vi "RDS Serial Handler Read.vi"(8 "error in (no error)":errorcluster, 11 "RDS Serial Instrument in":refnum<class "RDS Serial Instrument.lvclass">) -> (0 "error out":errorcluster, 1 "Data Valid?":bool, 2 "RDS Serial Frame out":refnum<class "RDS Serial Frame.lvclass">, 3 "RDS Serial Instrument out":refnum<class "RDS Serial Instrument.lvclass">)   [LabVIEW 2015, in "RDS Serial Handler.lvlib" / "RDS Serial Instrument.lvclass"]
doc: "Neat little program that reads the serial port and looks for a set of termination characters. The reason for this is that labview's serial functions only accept ONE termination character, meaning that I'll have to do lots of work arounds to use it, so might as well make my own clean implementation. \n\nThis VI reads data from a serial port untill it times out or it finds the termination character."
uses:
  RDS Serial Instrument.lvclass
  RDS Serial Frame.lvclass
  RDS Serial Instrument.lvclass/RDS Serial Instrument.ctl
  RDS Serial Frame.lvclass/RDS Serial Frame.ctl
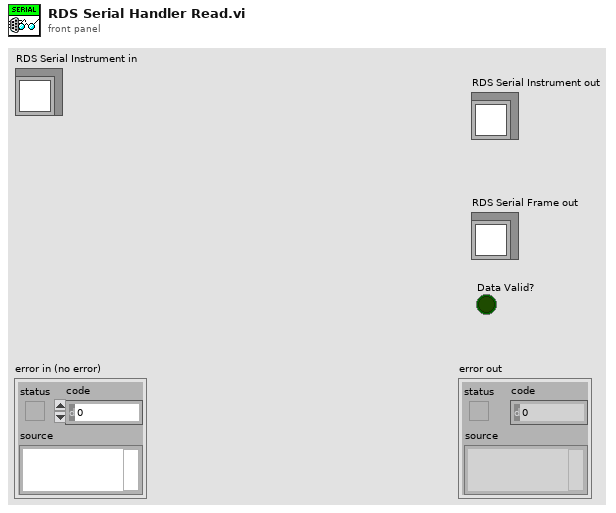
[diagram p1: front panel]
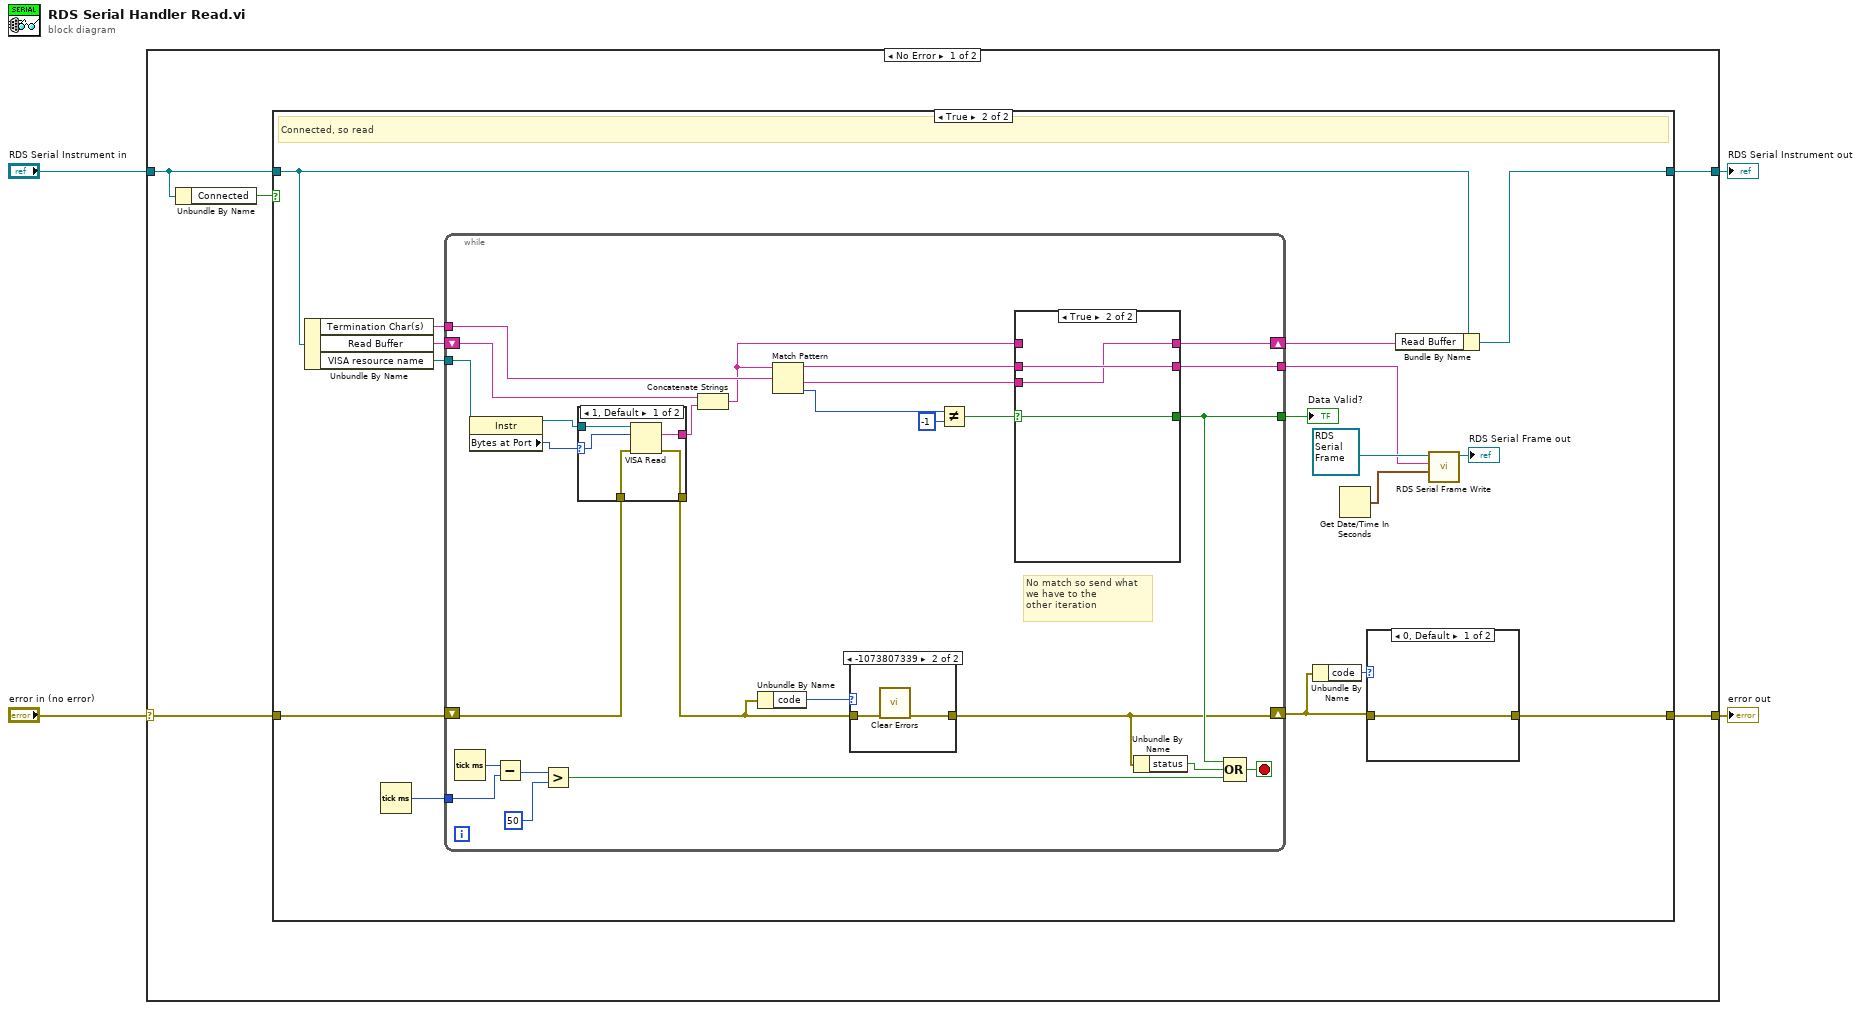
[diagram p0: block diagram]
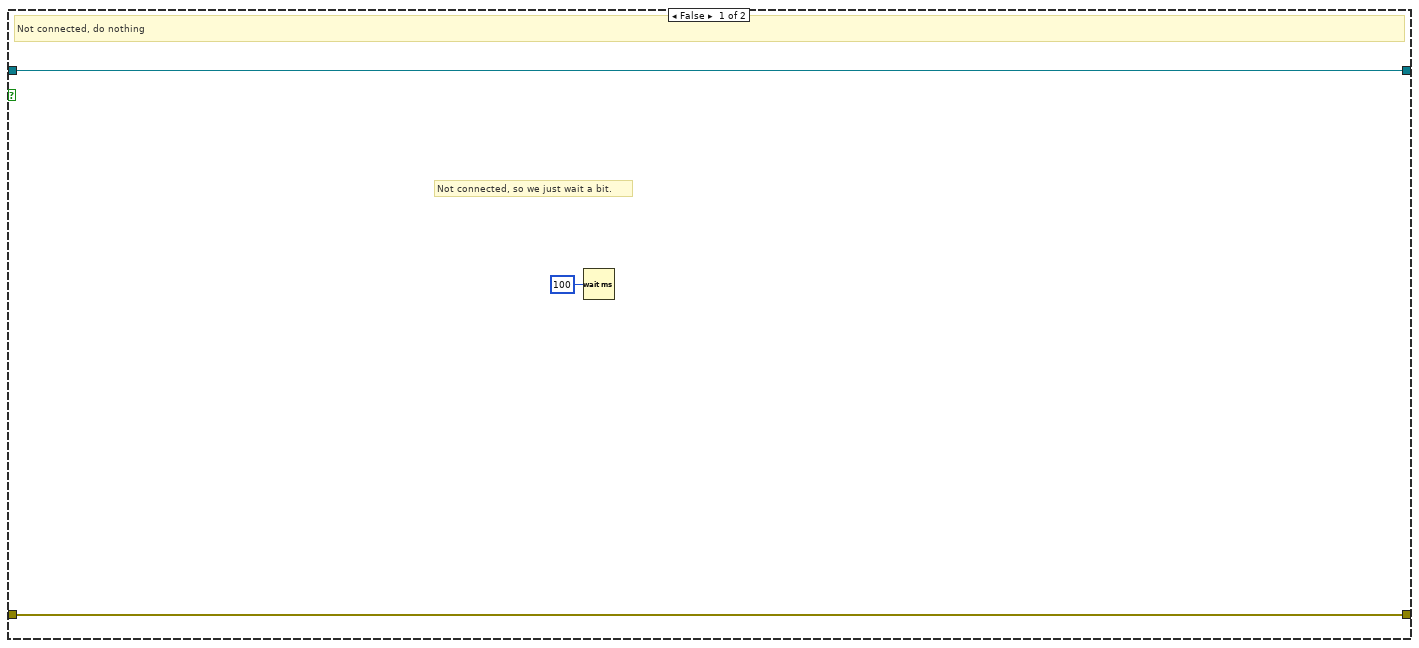
[diagram p2: hidden frame]
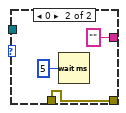
[diagram p3: hidden frame]
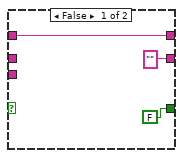
[diagram p4: hidden frame]
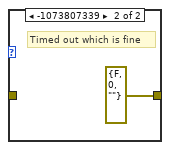
[diagram p6: hidden frame]
diagram:
  n1 = case shown="No Error" "error in (no error)" {
    selector: "error in (no error)" -> [w9 w75]
    tunnel: [w8 w75] -> w3
    tunnel: [w7 w74] -> w1
    tunnel: "RDS Serial Instrument in" -> [w6 w74]
    frame No Error {
      n2 = Unbundle By Name(w6) -> ("Connected"=w5:bool)
      n3 = case shown="True" w5 {
        tunnel: w9 -> [w11 w28]
        tunnel: [w11 w21] -> w8
        tunnel: w6 -> [w12 w20]
        tunnel: [w12 w19] -> w7
        frame False {
          # "Not connected, so we just wait a bit."
          # "Not connected, do nothing"
          n4 = Wait (ms)(milliseconds to wait=u32 100) -> ()  [unwired: 1 out]
        }
        frame True {
          # "Connected, so read"
          n5 = Unbundle By Name(w20) -> ("Termination Char(s)"=w25:string, "Read Buffer"=w27:string, "VISA resource name"=w26:refnum<visa-resource-name>)
          n6 = Tick Count (ms)() -> (millisecond timer value=w18:u32)
          n7 = while {
            tunnel: w26 -> [w38]
            tunnel: w25 -> [w51]
            tunnel: [w45] -> w24
            shift-right: [w39] -> w22
            shift-left: w28 -> [w54]
            shift-right: [w53] -> w16
            shift-left: w27 -> [w52]
            tunnel: [w50] -> w13
            tunnel: w18 -> [w48]
            stop <- w42 stop-if-true
            # "No match so send what\nwe have to the \nother iteration"
            n8 = Tick Count (ms)() -> (millisecond timer value=w49:u32)
            n9 = property class="Instr"(reference=w38) -> (reference out=w37:refnum<visa-resource-name>, "Bytes at Port"=w29:u32)  [unwired: 1 in, 1 out]
            n10 = Subtract(x=w49, y=w48) -> (x-y=w47:u32)
            n11 = Greater?(x=w47, y=u32 50) -> (0:w44:bool)
            n12 = case shown="1, Default" w29 {
              selector: w29 -> [w55 _]
              tunnel: w54 -> [w59 w60]
              tunnel: [w58 w60] -> w41
              tunnel: w37 -> [w57 _]
              tunnel: [w56 "" ("read buffer")] -> w30
              frame 1, Default {
                n13 = VISA Read(VISA resource name=w57, byte count=w55, error in (no error)=w59) -> (read buffer=w56:string, error out=w58:errorcluster)  [unwired: 2 out]
              }
              frame 0 {
                n14 = Wait (ms)(milliseconds to wait=u32 5) -> ()  [unwired: 1 out]
              }
            }
            n15 = Concatenate Strings(w52, w30) -> (w32:string)
            n16 = Unbundle By Name(w41) -> ("code"=w40:i32)
            n17 = Match Pattern(string=w32, regular expression=w51) -> (before substring=w34:string, after substring=w33:string, offset past match=w36:i32)  [unwired: 1 in, 1 out]
            n18 = case shown="-1073807339" w40 {
              tunnel: w41 -> [w69 w71]
              tunnel: [w69 w70] -> w39
              frame 0, Default {
              }
              frame -1073807339 {
                n19 = call <vilib>:"Clear Errors.vi"("error in (no error)"=w71) -> ("error out"=w70:errorcluster)  [unwired: 5 in, 1 out]
              }
            }
            n20 = Not Equal?(x=w36, y=-1) -> (x != y?=w31:bool)
            n21 = case shown="True" w31 {
              selector: w31 -> [_ w66]
              tunnel: w34 -> [_ w68]
              tunnel: ["" w68] -> w50
              tunnel: [w65 w67] -> w53
              tunnel: w33 -> [_ w67]
              tunnel: w32 -> [w65 _]
              tunnel: [FALSE w66] -> w45
              frame False {
              }
              frame True {
              }
            }
            n22 = Unbundle By Name(w39) -> ("status"=w43:bool)
            n23 = Compound Arithmetic op=OR(w45, w43, w44) -> (w42:bool)
          }
          "Data Valid?" <- w24
          n24 = Unbundle By Name(w22) -> ("code"=w23:i32)
          n25 = Get Date/Time In Seconds() -> (seconds since 1Jan1904=w15:timestamp)
          n26 = case shown="0, Default" w23 {
            tunnel: w22 -> [w72 _]
            tunnel: [w72 errorcluster {"status"=FALSE, "code"=0, "source"=""} ("error IO")] -> w21
            frame 0, Default {
            }
            frame -1073807339 {
              # "Timed out which is fine"
            }
          }
          n27 = Bundle By Name(cluster=w20, "Read Buffer"=w16) -> (w19:refnum<class "RDS Serial Instrument.lvclass">)
          n28 = call "RDS Serial Frame Write.vi"("Time Stamp"=w15, "Serial String"=w13, "RDS Serial Frame in"=refnum<class "RDS Serial Frame.lvclass"> refnum ("RDS Serial Handler.lvlib:RDS Serial Frame.lvclass")) -> ("RDS Serial Frame out"=→"RDS Serial Frame out":refnum<class "RDS Serial Frame.lvclass">)  [unwired: 7 in, 1 out]
        }
      }
    }
    frame Error {
    }
  }
  "error out" <- w3
  "RDS Serial Instrument out" <- w1
